vi "holdangle.vi"(9 "input":dbl, 10 "activate":bool) -> (2 "output":dbl)   [LabVIEW 2020]
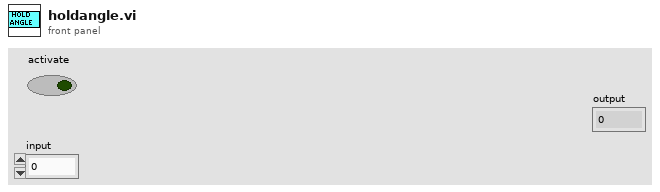
[diagram p1: front panel]
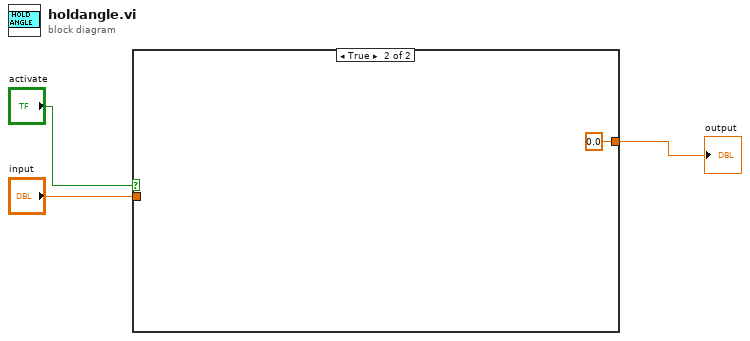
[diagram p0: block diagram]
diagram:
  n1 = case shown="True" "activate" {
    tunnel: [w4 0.0 ("input")] -> w2
    tunnel: "input" -> [w4 _]
    frame False {
    }
    frame True {
    }
  }
  "output" <- w2
